vi "RS232 - IIC_H3C QSFP+加密.vi"(0 "VISA resource name":refnum<visa-resource-name>="COM1", 1 "Function":T1(ring)=enum."Read From EEPROM1", 2 "Select channel":u32 max=1, 3 "input_psw":u8[](array[numeric])=[48, 97, 57, 122] format="%.0x", 4 "Data to write":u8[](array[numeric])=[1, 2, 3, 4, 5, 6, 7, 76, 117, 120, 115, 104, 97, 114, 101, 32, 83, 90, 32, 32, 32, 32, 32, 32, 0, 0, 9, 58, 88, 88, 88, 88, 88, 45, 88, 88, 88, 88, 32, 32, 32, 32, 32, 32, 69, 32, 32, 32, 0, 0, 0, 0, 0, 56, 56, 56, 56, 56, 56, 56, 56, 56, 56, 32, 32, 32, 32, 32, 32, 48, 56, 48, 51, 51, 0, 0, 0, 0, 0, 46, 46, 46, 46, 46, 46, 46, 46, 46, 46, 32, 105, 50, 99, 32, 116, 101, 115, 116, 105, 110, 103, 45, 45, 45, 45, 45, 32, 99, 111, 109, 112, 108, 101, 116, 101, 100, 32, 97, 110, 100, 32, 115, 117, 99, 99, 101, 115, 115, 102, 117, 108] format="%x", 5 "Error in":errorcluster) -> (12 "3PagesEqual0":bool, 13 "EEPROM read data":string[][](array[string]), 14 "Duplicate VISA resource name":refnum<visa-resource-name>, 15 "Read Data":string, 16 "Data from Read":u8[](array[numeric])=[255, 255, 255, 255, 255, 255, 255, 255, 255, 255, 255, 255, 255, 255, 255, 255, 255, 255, 255, 255, 255, 82, 101, 118, 49, 46, 49, 255, 255, 255, 255, 255, 255, 255, 255, 255, 255, 255, 255, 255, 255, 255, 255, 255, 255, 255, 255, 255, 255, 255, 255, 255, 255, 255, 255, 255, 255, 255, 255, 255, 255, 255, 255, 255, 255, 255, 255, 255, 255, 255, 255, 255, 255, 255, 255, 255, 255, 255, 255, 255, 255, 255, 255, 255, 255, 255, 255, 255, 255, 255, 255, 255, 255, 255, 255, 255, 255, 255, 255, 255, 255, 255, 255, 255, 255, 255, 255, 255, 255, 255, 255, 255, 255, 255, 255, 255, 255, 255, 255, 255, 255, 255, 255, 255, 255, 255, 255, 255, 255, 255, 255, 255, 255, 255, 255, 255, 255, 255, 255, 255, 255, 255, 255, 255, 255, 255, 255, 255, 255, 82, 101, 118, 49, 46, 49, 255, 255, 255, 255, 255, 255, 255, 255, 255, 255, 255, 255, 255, 255, 255, 255, 255, 255, 255, 255, 255, 255, 255, 255, 255, 255, 255, 255, 255, 255, 255, 255, 255, 255, 255, 255, 255, 255, 255, 255, 255, 255, 255, 255, 255, 255, 255, 255, 255, 255, 255, 255, 255, 255, 255, 255, 255, 255, 255, 255, 255, 255, 255, 255, 255, 255, 255, 255, 255, 255, 255, 255, 255, 255, 255, 255, 255, 255, 255, 255, 255, 255, 255, 255, 255, 255, 255, 255, 255, 255, 255, 255, 255, 255, 255, 255, 255, 255, 255, 255, 255, 255] format="%x", 17 "Message":string, 18 "status":bool=TRUE, 19 "error out":errorcluster={"status"=FALSE, "code"=1073676294, "source"="RS232 - IIC_H3C QSFP+加密.vi中的VISA读取"})   [LabVIEW 2011]
uses:
  <vilib>/Instr/_visa.llb/VISA Configure Serial Port (Instr).vi
panel:
  out "bools":bool[](array[boolean])
  out "x = y?":bool
  out "arrya":u8[][](array[numeric]) format="%.0x"
  in  "Mode":u32(ring) items=["0~EasyI2C", "1~TimingI2C"]
  # "RS232-I2C Writting and Reading"
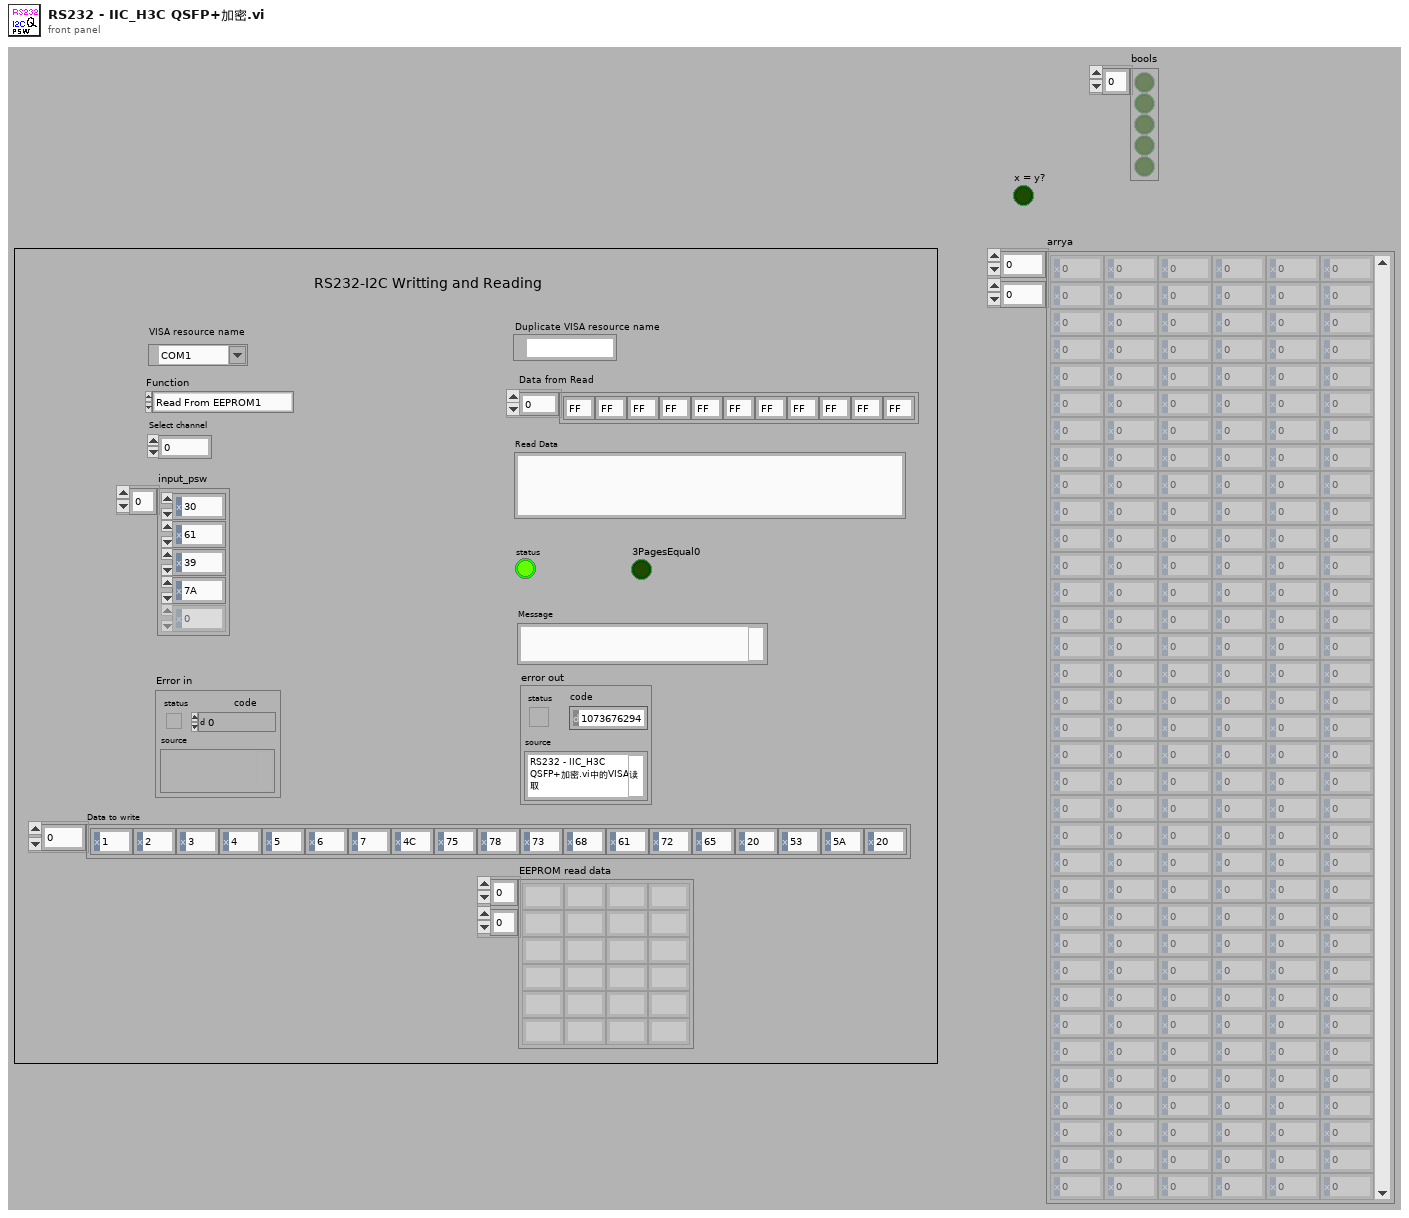
[diagram p1: front panel]
types:
  T1 = enum16{"Write to EEPROM", "Read From EEPROM", "Read From EEPROM1"}
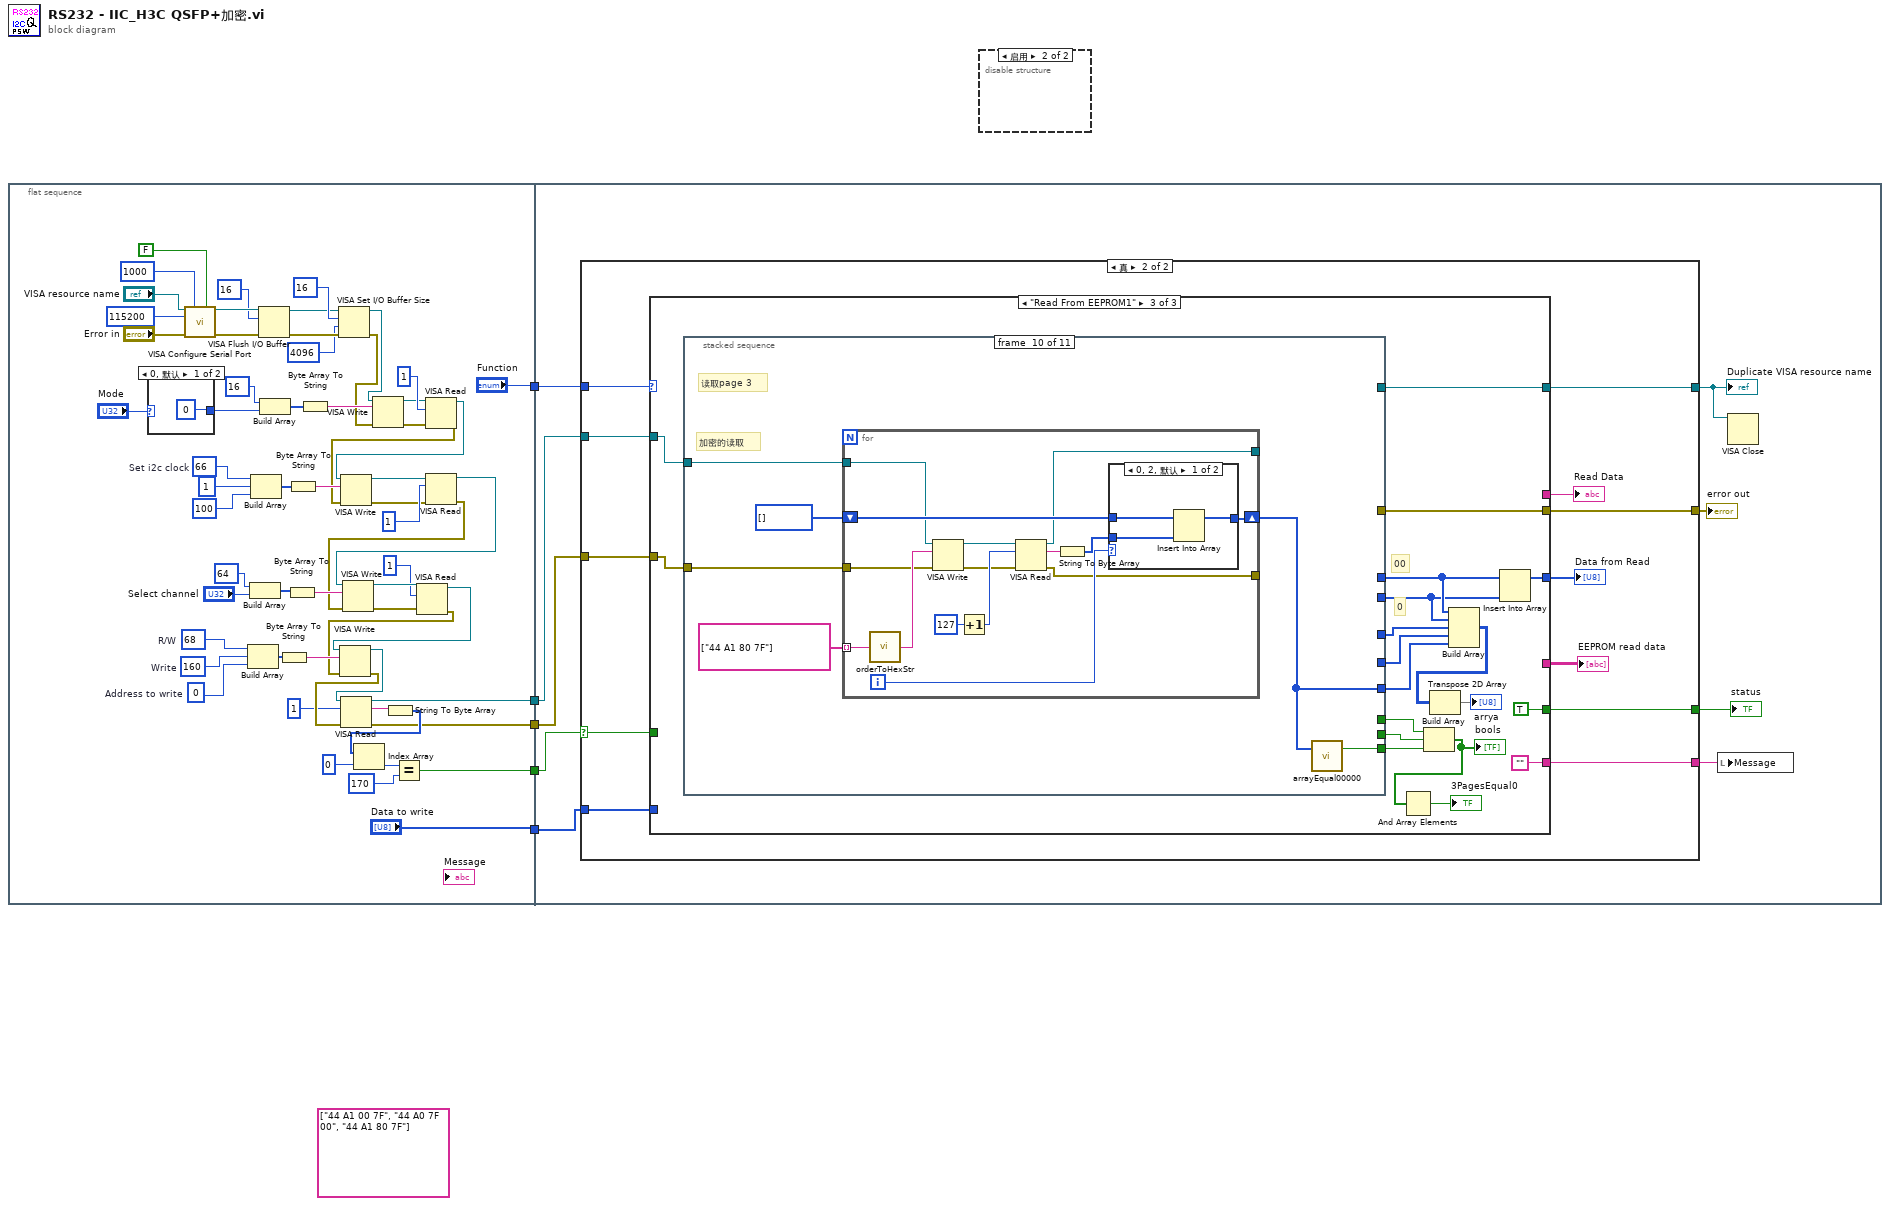
[diagram p0: block diagram]
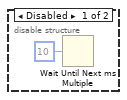
[diagram p2: hidden frame]
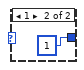
[diagram p3: hidden frame]
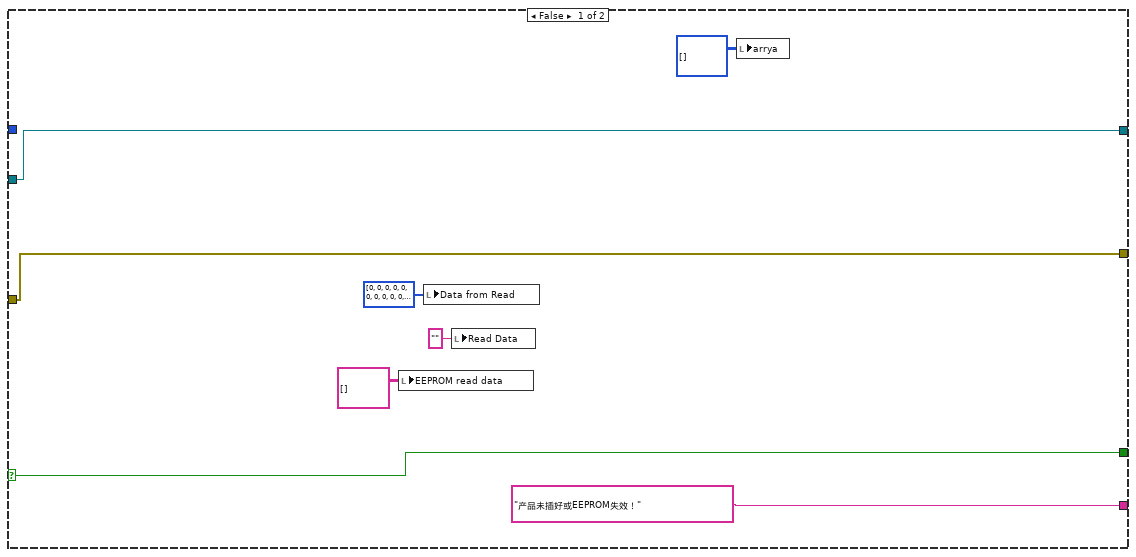
[diagram p4: hidden frame]
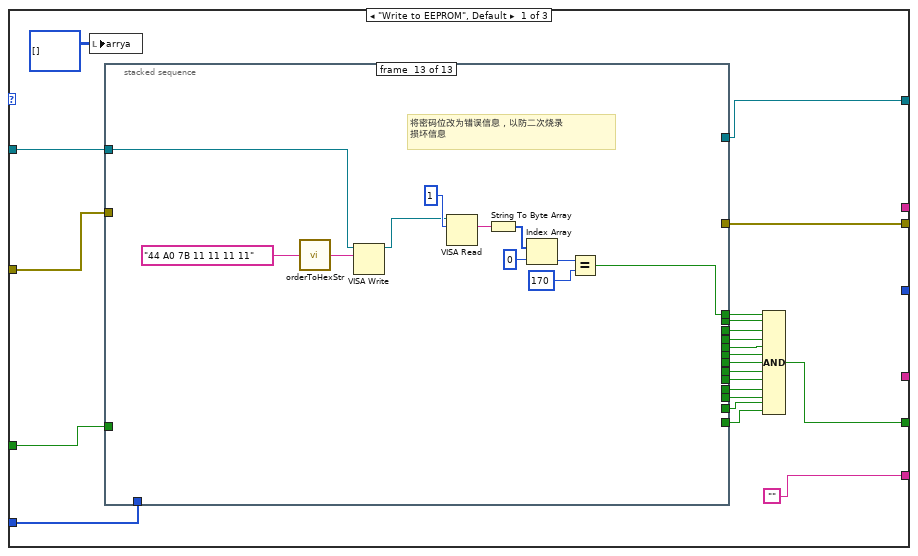
[diagram p5: hidden frame]
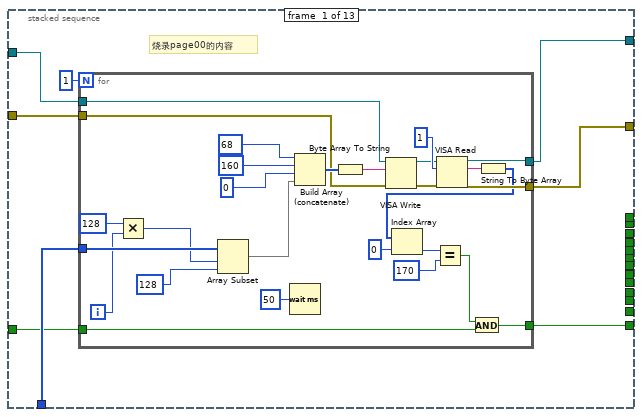
[diagram p6: hidden frame]
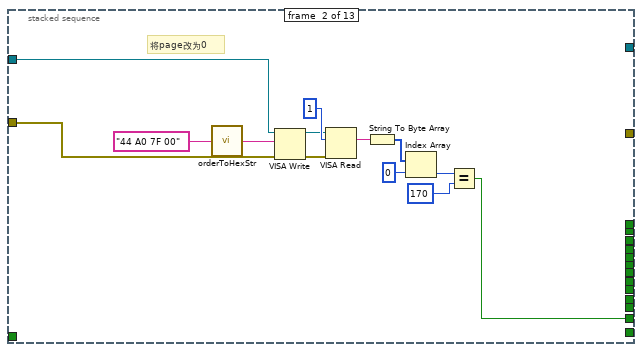
[diagram p7: hidden frame]
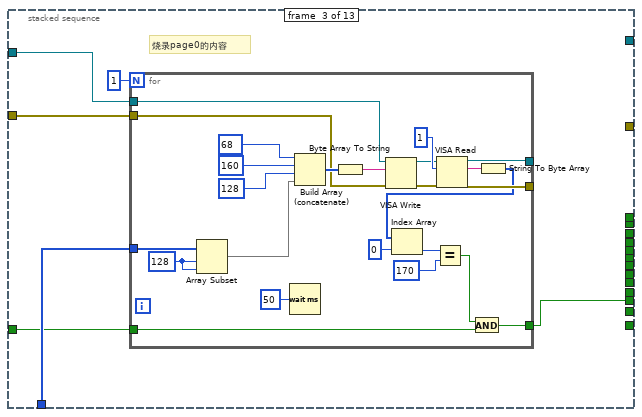
[diagram p8: hidden frame]
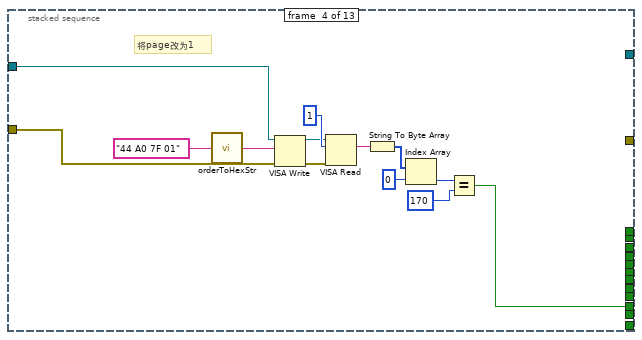
[diagram p9: hidden frame]
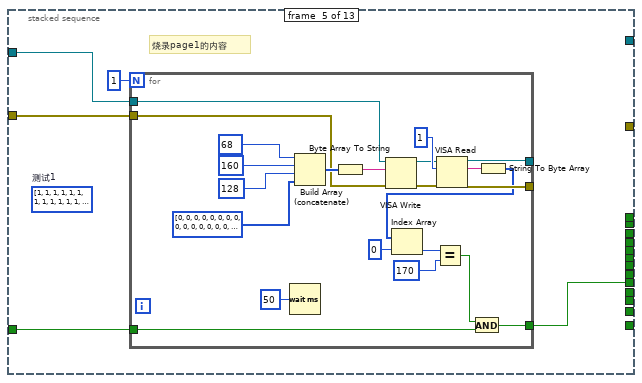
[diagram p10: hidden frame]
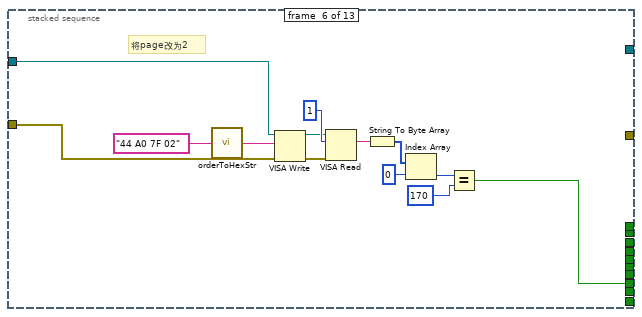
[diagram p11: hidden frame]
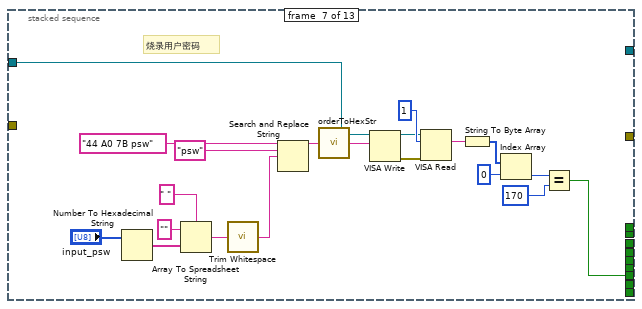
[diagram p12: hidden frame]
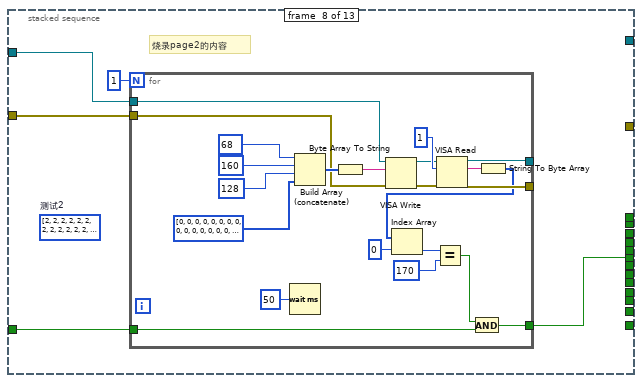
[diagram p13: hidden frame]
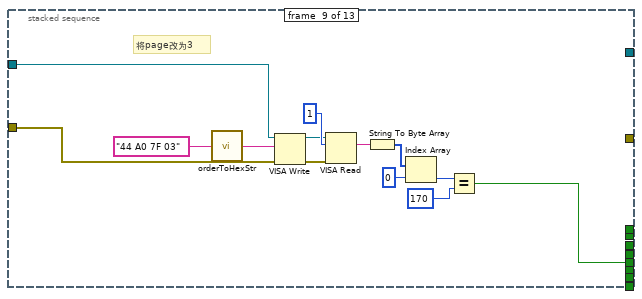
[diagram p14: hidden frame]
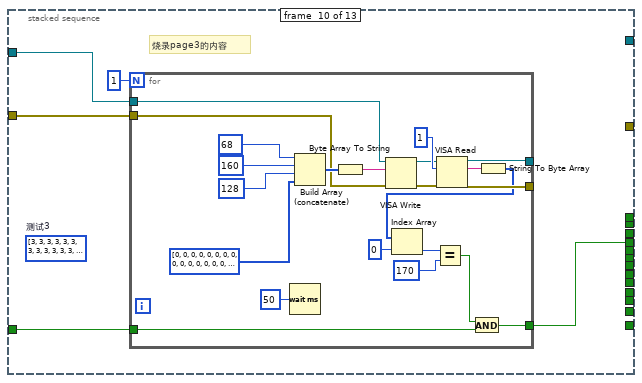
[diagram p15: hidden frame]
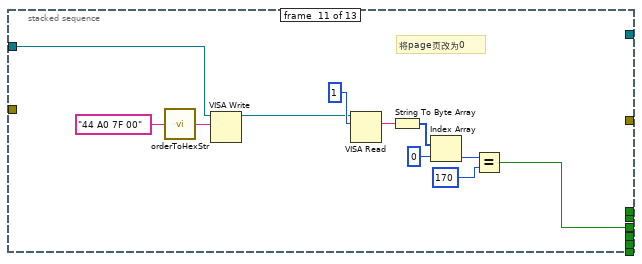
[diagram p16: hidden frame]
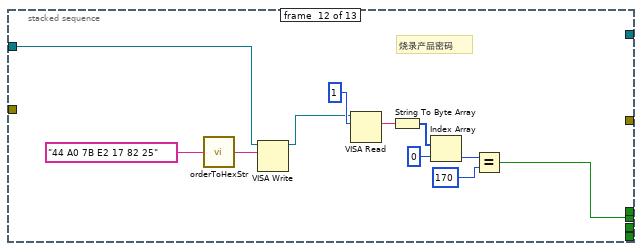
[diagram p17: hidden frame]
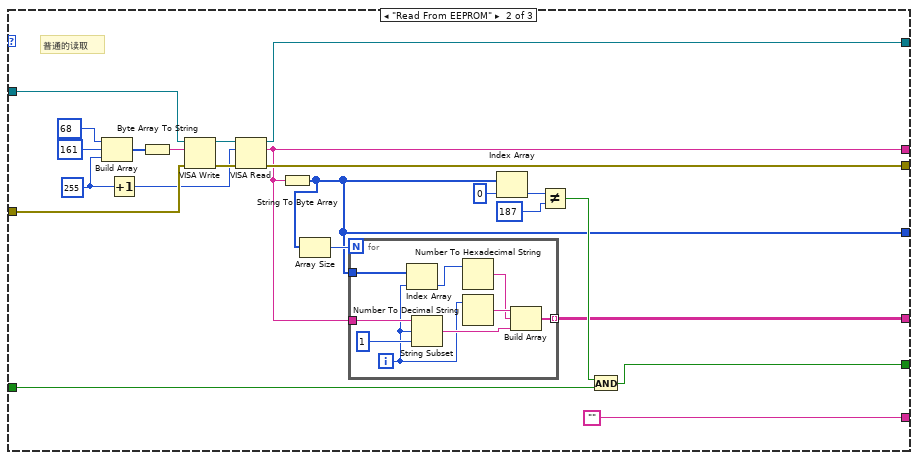
[diagram p18: hidden frame]
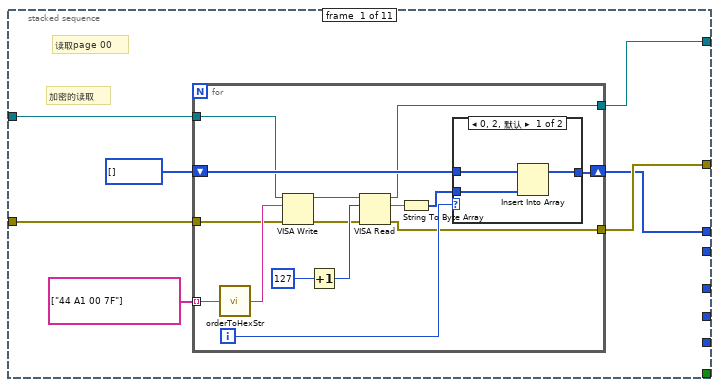
[diagram p19: hidden frame]
diagram:
  (unwired) string[] ["44 A1 00 7F", "44 A0 7F 00", "44 A1 80 7F"]
  n1 = flat-sequence {
    tunnel: [w27] -> w5
    tunnel: [w26] -> w4
    tunnel: [w25] -> w3
    tunnel: ["Function"] -> w2
    tunnel: ["Data to write"] -> w1
    tunnel: w5 -> [w77]
    tunnel: w4 -> [w76]
    tunnel: w3 -> [w75]
    tunnel: w2 -> [w74]
    tunnel: w1 -> [w73]
    frame #0 {
      w31 = u32 0  # Address to write
      w35 = u32 160  # Write
      w33 = u32 68  # R/W
      w48 = u32 66  # Set i2c clock
      n2 = case shown="0, 默认" "Mode" {
        tunnel: [u32 0 ("channel") u32 1 ("channel")] -> w54
        frame 0, Default {
        }
        frame 1 {
        }
      }
      n3 = call-poly "VISA Configure Serial Port"("VISA resource name"="VISA resource name", "timeout (10sec)"=u32 1000 ("timeout"), "Enable Termination\nChar (T)"=FALSE ("Enable Termination\nChar (T)"), "baud rate (9600)"=u32 115200 ("baud rate"), "error in (no error)"="Error in") -> ("VISA resource name out"=w66:refnum<visa-resource-name>, "error out"=w41:errorcluster)  [unwired: 9 in]
      n4 = Build Array(w33, w35, w31) -> (w34:u32[])
      n5 = Build Array(u32 64 ("size (0)"), "Select channel") -> (w52:u32[])
      n6 = Build Array(w48, u32 1 ("size (0)"), u32 100 ("size (0)")) -> (w47:u32[])
      n7 = VISA Flush I/O Buffer(VISA resource name=w66, mask (16)=u16 16, error in (no error)=w41) -> (VISA resource name out=w63:refnum<visa-resource-name>, error out=w62:errorcluster)
      n8 = Build Array(u32 16 ("size (0)"), w54) -> (w53:u32[])
      n9 = Byte Array To String(unsigned byte array=w34) -> (string=w38:string)
      n10 = Byte Array To String(unsigned byte array=w52) -> (string=w44:string)
      n11 = Byte Array To String(unsigned byte array=w47) -> (string=w43:string)
      n12 = Byte Array To String(unsigned byte array=w53) -> (string=w56:string)
      n13 = VISA Set I/O Buffer Size(VISA resource name=w63, mask (16)=u16 16, size (4096)=u32 4096 ("size (0)"), error in (no error)=w62) -> (VISA resource name out=w57:refnum<visa-resource-name>, error out=w40:errorcluster)
      n14 = VISA Write(VISA resource name=w57, write buffer=w56, error in (no error)=w40) -> (VISA resource name out=w19:refnum<visa-resource-name>, error out=w18:errorcluster)  [unwired: 1 out]
      n15 = VISA Read(VISA resource name=w19, byte count=u32 1, error in (no error)=w18) -> (VISA resource name out=w17:refnum<visa-resource-name>, error out=w14:errorcluster)  [unwired: 2 out]
      n16 = VISA Write(VISA resource name=w17, write buffer=w43, error in (no error)=w14) -> (VISA resource name out=w16:refnum<visa-resource-name>, error out=w13:errorcluster)  [unwired: 1 out]
      n17 = VISA Read(VISA resource name=w16, byte count=u32 1, error in (no error)=w13) -> (VISA resource name out=w15:refnum<visa-resource-name>, error out=w12:errorcluster)  [unwired: 2 out]
      n18 = VISA Write(VISA resource name=w15, write buffer=w44, error in (no error)=w12) -> (VISA resource name out=w11:refnum<visa-resource-name>, error out=w10:errorcluster)  [unwired: 1 out]
      n19 = VISA Read(VISA resource name=w11, byte count=u32 1, error in (no error)=w10) -> (VISA resource name out=w8:refnum<visa-resource-name>, error out=w7:errorcluster)  [unwired: 2 out]
      n20 = VISA Write(VISA resource name=w8, write buffer=w38, error in (no error)=w7) -> (VISA resource name out=w32:refnum<visa-resource-name>, error out=w39:errorcluster)  [unwired: 1 out]
      n21 = VISA Read(VISA resource name=w32, byte count=u32 1, error in (no error)=w39) -> (VISA resource name out=w26:refnum<visa-resource-name>, read buffer=w37:string, error out=w25:errorcluster)  [unwired: 1 out]
      n22 = String To Byte Array(string=w37) -> (unsigned byte array=w28:u8[])
      n23 = Index Array(array=w28, index=0) -> (element=w30:u8)
      n24 = Equal?(x=w30, y=u32 170 ("size (0)")) -> (x = y?=w27:bool)
    }
    frame #1 {
      n25 = case shown="真" w77 {
        selector: w77 -> [w82 w93]
        tunnel: w76 -> [w84 w97]
        tunnel: w75 -> [w85 w96]
        tunnel: w74 -> [_ w95]
        tunnel: w73 -> [_ w94]
        tunnel: [w85 w92] -> w70
        tunnel: [w84 w91] -> w69
        tunnel: ["产品未插好或EEPROM失效！" ("message") w90] -> w72
        tunnel: [w82 w86] -> w71
        frame False {
          n26 = local write "EEPROM read data"(string[][] [] ("EEPROM read data")) -> ()
          n27 = local write "Data from Read"(i32[] [0, 0, 0, 0, 0, 0, 0, 0, 0, 0, 0, 0, 0, 0, 0, 0, 0, 0, 0, 0, 0, 0, 0, 0, 0, 0, 0, 0, 0, 0, 0, 0, 0, 0, 0, 0, 0, 0, 0, 0, 0, 0, 0, 0, 0, 0, 0, 0, 0, 0, 0, 0, 0, 0, 0, 0, 0, 0, 0, 0, 0, 0, 0, 0, 0, 0, 0, 0, 0, 0, 0, 0, 0, 0, 0, 0, 0, 0, 0, 0, 0, 0, 0, 0, 0, 0, 0, 0, 0, 0, 0, 0, 0, 0, 0, 0, 0, 0, 0, 0, 0, 0, 0, 0, 0, 0, 0, 0, 0, 0, 0, 0, 0, 0, 0, 0, 0, 0, 0, 0, 0, 0, 0, 0, 0, 0, 0, 0, 0, 0, 0, 0, 0, 0, 0, 0, 0, 0, 0, 0, 0, 0, 0, 0, 0, 0, 0, 0, 0, 0, 0, 0, 0, 0, 0, 0, 0, 0, 0, 0, 0, 0, 0, 0, 0, 0, 0, 0, 0, 0, 0, 0, 0, 0, 0, 0, 0, 0, 0, 0, 0, 0, 0, 0, 0, 0, 0, 0, 0, 0, 0, 0, 0, 0, 0, 0, 0, 0, 0, 0, 0, 0, 0, 0, 0, 0, 0, 0, 0, 0, 0, 0, 0, 0, 0, 0, 0, 0, 0, 0, 0, 0, 0, 0, 0, 0, 0, 0, 0, 0, 0, 0, 0, 0, 0, 0, 0, 0, 0, 0, 0, 0, 0, 0, 0, 0, 0, 0, 0, 0, 0, 0, 0, 0, 0, 0] ("Data from Read")) -> ()
          n28 = local write "Read Data"("" ("Read Data")) -> ()
          n29 = local write "arrya"(u8[][] [] ("arrya")) -> ()
        }
        frame True {
          n30 = case shown="\"Read From EEPROM1\"" w95 {
            tunnel: w97 -> [w119 w393 w419]
            tunnel: w96 -> [w118 w392 w417]
            tunnel: w94 -> [w117 _ _]
            tunnel: [w114 w371 w418] -> w91
            tunnel: [w116 w385 w416] -> w92
            tunnel: w93 -> [w113 w377 _]
            tunnel: ["" ("Message") "" ("Message") "" ("Message")] -> w90
            tunnel: [w101 w375 TRUE] -> w86
            tunnel: [_ w374 _] -> w89
            tunnel: [_ w373 w415] -> w88
            tunnel: [_ w372 _] -> w87
            frame "Write to EEPROM", Default {
              n31 = local write "arrya"(u8[][] [] ("arrya")) -> ()
              n32 = stacked-sequence {
                tunnel: w119 -> [w127 w159 w173 w202 w215 w242 w261 w275 w302 w315 w339 w351 w362]
                tunnel: w118 -> [w126 w158 w172 w201 w214 w241 _ w274 w301 w314 _ _ _]
                tunnel: w117 -> [w125 _ w171 _ _ _ _ _ _ _ _ _ _]
                tunnel: [w123 _ _ _ _ _ _ _ _ _ _ _ _] -> w116
                tunnel: [w124 _ _ _ _ _ _ _ _ _ _ _ _] -> w114
                tunnel: w113 -> [w122 _ w170 _ w213 _ _ w273 _ w313 _ _ _]
                tunnel: [w121 _ _ _ _ _ _ _ _ _ _ _ _] -> w102
                tunnel: [_ w155 _ _ _ _ _ _ _ _ _ _ _] -> w103
                tunnel: [_ _ w168 _ _ _ _ _ _ _ _ _ _] -> w104
                tunnel: [_ _ _ w198 _ _ _ _ _ _ _ _ _] -> w105
                tunnel: [_ _ _ _ w211 _ _ _ _ _ _ _ _] -> w106
                tunnel: [_ _ _ _ _ w238 _ _ _ _ _ _ _] -> w107
                tunnel: [_ _ _ _ _ _ w251 _ _ _ _ _ _] -> w108
                tunnel: [_ _ _ _ _ _ _ w271 _ _ _ _ _] -> w109
                tunnel: [_ _ _ _ _ _ _ _ w298 _ _ _ _] -> w110
                tunnel: [_ _ _ _ _ _ _ _ _ w311 _ _ _] -> w111
                tunnel: [_ _ _ _ _ _ _ _ _ _ w341 _ _] -> w112
                tunnel: [_ _ _ _ _ _ _ _ _ _ _ w349 _] -> w100
                tunnel: [_ _ _ _ _ _ _ _ _ _ _ _ w360] -> w99
                frame #0 {
                  # "烧录page00的内容"
                  n33 = for {
                    N: 1 -> [_]
                    tunnel: w127 -> [w150]
                    tunnel: w125 -> [w133]
                    tunnel: w126 -> [w149]
                    tunnel: [w144] -> w123
                    tunnel: [w142] -> w124
                    tunnel: w122 -> [w137]
                    tunnel: [w136] -> w121
                    i -> [w130]
                    n34 = Multiply(x=128, y=w130) -> (x*y=w128:i32)
                    n35 = Array Subset(array=w133, index=w128, length=128 ("长度")) -> (w131:u8[])
                    n36 = Wait (ms)(milliseconds to wait=u32 50 ("等待时间（毫秒）")) -> ()  [unwired: 1 out]
                    n37 = Build Array (concatenate)(u32 68 ("Write data"), u32 160 ("size (0)"), u32 0 ("元素"), w131) -> (w153:u32[])
                    n38 = Byte Array To String(unsigned byte array=w153) -> (string=w151:string)
                    n39 = VISA Write(VISA resource name=w150, write buffer=w151, error in (no error)=w149) -> (VISA resource name out=w145:refnum<visa-resource-name>, error out=w143:errorcluster)  [unwired: 1 out]
                    n40 = VISA Read(VISA resource name=w145, byte count=u32 1, error in (no error)=w143) -> (VISA resource name out=w142:refnum<visa-resource-name>, read buffer=w141:string, error out=w144:errorcluster)  [unwired: 1 out]
                    n41 = String To Byte Array(string=w141) -> (unsigned byte array=w140:u8[])
                    n42 = Index Array(array=w140, index=0) -> (element=w139:u8)
                    n43 = Equal?(x=w139, y=u32 170 ("size (0)")) -> (x = y?=w138:bool)
                    n44 = And(x=w138, y=w137) -> (x .and. y?=w136:bool)
                  }
                }
                frame #1 {
                  # "将page改为0"
                  n45 = call "orderToHexStr.vi"("I"="44 A0 7F 00") -> ("O"=w156:string)
                  n46 = VISA Write(VISA resource name=w159, write buffer=w156, error in (no error)=w158) -> (VISA resource name out=w164:refnum<visa-resource-name>, error out=w163:errorcluster)  [unwired: 1 out]
                  n47 = VISA Read(VISA resource name=w164, byte count=u32 1, error in (no error)=w163) -> (read buffer=w162:string)  [unwired: 3 out]
                  n48 = String To Byte Array(string=w162) -> (unsigned byte array=w161:u8[])
                  n49 = Index Array(array=w161, index=0) -> (element=w160:u8)
                  n50 = Equal?(x=w160, y=u32 170 ("size (0)")) -> (x = y?=w155:bool)
                }
                frame #2 {
                  # "烧录page0的内容"
                  n51 = for {
                    N: 1 -> [_]
                    tunnel: w173 -> [w193]
                    tunnel: w171 -> [w176]
                    tunnel: w172 -> [w192]
                    tunnel: [w187] -> _
                    tunnel: [w185] -> _
                    tunnel: w170 -> [w180]
                    tunnel: [w179] -> w168
                    w175 = 128 ("索引")
                    n52 = Array Subset(array=w176, index=w175, length=w175) -> (w174:u8[])
                    n53 = Wait (ms)(milliseconds to wait=u32 50 ("等待时间（毫秒）")) -> ()  [unwired: 1 out]
                    n54 = Build Array (concatenate)(u8 68 ("Write data"), u8 160 ("size (0)"), u8 128 ("元素"), w174) -> (w196:u8[])
                    n55 = Byte Array To String(unsigned byte array=w196) -> (string=w194:string)
                    n56 = VISA Write(VISA resource name=w193, write buffer=w194, error in (no error)=w192) -> (VISA resource name out=w188:refnum<visa-resource-name>, error out=w186:errorcluster)  [unwired: 1 out]
                    n57 = VISA Read(VISA resource name=w188, byte count=u32 1, error in (no error)=w186) -> (VISA resource name out=w185:refnum<visa-resource-name>, read buffer=w184:string, error out=w187:errorcluster)  [unwired: 1 out]
                    n58 = String To Byte Array(string=w184) -> (unsigned byte array=w183:u8[])
                    n59 = Index Array(array=w183, index=0) -> (element=w182:u8)
                    n60 = Equal?(x=w182, y=u32 170 ("size (0)")) -> (x = y?=w181:bool)
                    n61 = And(x=w181, y=w180) -> (x .and. y?=w179:bool)
                  }
                }
                frame #3 {
                  # "将page改为1"
                  n62 = call "orderToHexStr.vi"("I"="44 A0 7F 01") -> ("O"=w199:string)
                  n63 = VISA Write(VISA resource name=w202, write buffer=w199, error in (no error)=w201) -> (VISA resource name out=w207:refnum<visa-resource-name>, error out=w206:errorcluster)  [unwired: 1 out]
                  n64 = VISA Read(VISA resource name=w207, byte count=u32 1, error in (no error)=w206) -> (read buffer=w205:string)  [unwired: 3 out]
                  n65 = String To Byte Array(string=w205) -> (unsigned byte array=w204:u8[])
                  n66 = Index Array(array=w204, index=0) -> (element=w203:u8)
                  n67 = Equal?(x=w203, y=u32 170 ("size (0)")) -> (x = y?=w198:bool)
                }
                frame #4 {
                  (unwired) u8[] [1, 1, 1, 1, 1, 1, 1, 1, 1, 1, 1, 1, 1, 1, 1, 1, 1, 1, 1, 1, 1, 1, 1, 1, 1, 1, 1, 1, 1, 1, 1, 1, 1, 1, 1, 1, 1, 1, 1, 1, 1, 1, 1, 1, 1, 1, 1, 1, 1, 1, 1, 1, 1, 1, 1, 1, 1, 1, 1, 1, 1, 1, 1, 1, 1, 1, 1, 1, 1, 1, 1, 1, 1, 1, 1, 1, 1, 1, 1, 1, 1, 1, 1, 1, 1, 1, 1, 1, 1, 1, 1, 1, 1, 1, 1, 1, 1, 1, 1, 1, 1, 1, 1, 1, 1, 1, 1, 1, 1, 1, 1, 1, 1, 1, 1, 1, 1, 1, 1, 1, 1, 1, 1, 1, 1, 1, 1, 1]  # 测试1
                  # "烧录page1的内容"
                  n68 = for {
                    N: 1 -> [_]
                    tunnel: w215 -> [w233]
                    tunnel: w214 -> [w232]
                    tunnel: [w227] -> _
                    tunnel: [w225] -> _
                    tunnel: w213 -> [w220]
                    tunnel: [w219] -> w211
                    n69 = Wait (ms)(milliseconds to wait=u32 50 ("等待时间（毫秒）")) -> ()  [unwired: 1 out]
                    n70 = Build Array (concatenate)(u8 68 ("Write data"), u8 160 ("size (0)"), u8 128 ("元素"), u8[] [0, 0, 0, 0, 0, 0, 0, 0, 0, 0, 0, 0, 0, 0, 0, 0, 0, 0, 0, 0, 0, 0, 0, 0, 0, 0, 0, 0, 0, 0, 0, 0, 0, 0, 0, 0, 0, 0, 0, 0, 0, 0, 0, 0, 0, 0, 0, 0, 0, 0, 0, 0, 0, 0, 0, 0, 0, 0, 0, 0, 0, 0, 0, 0, 0, 0, 0, 0, 0, 0, 0, 0, 0, 0, 0, 0, 0, 0, 0, 0, 0, 0, 0, 0, 0, 0, 0, 0, 0, 0, 0, 0, 0, 0, 0, 0, 0, 0, 0, 0, 0, 0, 0, 0, 0, 0, 0, 0, 0, 0, 0, 0, 0, 0, 0, 0, 0, 0, 0, 0, 0, 0, 0, 0, 0, 0, 0, 0]) -> (w236:u8[])
                    n71 = Byte Array To String(unsigned byte array=w236) -> (string=w234:string)
                    n72 = VISA Write(VISA resource name=w233, write buffer=w234, error in (no error)=w232) -> (VISA resource name out=w228:refnum<visa-resource-name>, error out=w226:errorcluster)  [unwired: 1 out]
                    n73 = VISA Read(VISA resource name=w228, byte count=u32 1, error in (no error)=w226) -> (VISA resource name out=w225:refnum<visa-resource-name>, read buffer=w224:string, error out=w227:errorcluster)  [unwired: 1 out]
                    n74 = String To Byte Array(string=w224) -> (unsigned byte array=w223:u8[])
                    n75 = Index Array(array=w223, index=0) -> (element=w222:u8)
                    n76 = Equal?(x=w222, y=u32 170 ("size (0)")) -> (x = y?=w221:bool)
                    n77 = And(x=w221, y=w220) -> (x .and. y?=w219:bool)
                  }
                }
                frame #5 {
                  # "将page改为2"
                  n78 = call "orderToHexStr.vi"("I"="44 A0 7F 02") -> ("O"=w239:string)
                  n79 = VISA Write(VISA resource name=w242, write buffer=w239, error in (no error)=w241) -> (VISA resource name out=w247:refnum<visa-resource-name>, error out=w246:errorcluster)  [unwired: 1 out]
                  n80 = VISA Read(VISA resource name=w247, byte count=u32 1, error in (no error)=w246) -> (read buffer=w245:string)  [unwired: 3 out]
                  n81 = String To Byte Array(string=w245) -> (unsigned byte array=w244:u8[])
                  n82 = Index Array(array=w244, index=0) -> (element=w243:u8)
                  n83 = Equal?(x=w243, y=u32 170 ("size (0)")) -> (x = y?=w238:bool)
                }
                frame #6 {
                  # "烧录用户密码"
                  n84 = Number To Hexadecimal String(2:"input_psw") -> (0:w258:string[])  [unwired: 1 in]
                  n85 = Array To Spreadsheet String(delimiter (Tab)=" " ("分隔符(Tab)"), array=w258, 3:"" ("格式字符串")) -> (spreadsheet string=w257:string)
                  n86 = call <vilib>:"Trim Whitespace.vi"("string"=w257) -> ("trimmed string"=w253:string)  [unwired: 1 in]
                  n87 = Search and Replace String(input string="44 A0 7B psw", search string="psw" ("搜索字符串"), replace string=w253) -> (result string=w252:string)  [unwired: 5 in, 3 out]
                  n88 = call "orderToHexStr.vi"("I"=w252) -> ("O"=w262:string)
                  n89 = VISA Write(VISA resource name=w261, write buffer=w262) -> (VISA resource name out=w267:refnum<visa-resource-name>, error out=w266:errorcluster)  [unwired: 1 in, 1 out]
                  n90 = VISA Read(VISA resource name=w267, byte count=u32 1, error in (no error)=w266) -> (read buffer=w265:string)  [unwired: 3 out]
                  n91 = String To Byte Array(string=w265) -> (unsigned byte array=w264:u8[])
                  n92 = Index Array(array=w264, index=0) -> (element=w263:u8)
                  n93 = Equal?(x=w263, y=u32 170 ("size (0)")) -> (x = y?=w251:bool)
                }
                frame #7 {
                  (unwired) u8[] [2, 2, 2, 2, 2, 2, 2, 2, 2, 2, 2, 2, 2, 2, 2, 2, 2, 2, 2, 2, 2, 2, 2, 2, 2, 2, 2, 2, 2, 2, 2, 2, 2, 2, 2, 2, 2, 2, 2, 2, 2, 2, 2, 2, 2, 2, 2, 2, 2, 2, 2, 2, 2, 2, 2, 2, 2, 2, 2, 2, 2, 2, 2, 2, 2, 2, 2, 2, 2, 2, 2, 2, 2, 2, 2, 2, 2, 2, 2, 2, 2, 2, 2, 2, 2, 2, 2, 2, 2, 2, 2, 2, 2, 2, 2, 2, 2, 2, 2, 2, 2, 2, 2, 2, 2, 2, 2, 2, 2, 2, 2, 2, 2, 2, 2, 2, 2, 2, 2, 2, 2, 2, 2, 2, 2, 2, 2, 2]  # 测试2
                  # "烧录page2的内容"
                  n94 = for {
                    N: 1 -> [_]
                    tunnel: w275 -> [w293]
                    tunnel: w274 -> [w292]
                    tunnel: [w287] -> _
                    tunnel: [w285] -> _
                    tunnel: w273 -> [w280]
                    tunnel: [w279] -> w271
                    n95 = Wait (ms)(milliseconds to wait=u32 50 ("等待时间（毫秒）")) -> ()  [unwired: 1 out]
                    n96 = Build Array (concatenate)(u8 68 ("Write data"), u8 160 ("size (0)"), u8 128 ("元素"), u8[] [0, 0, 0, 0, 0, 0, 0, 0, 0, 0, 0, 0, 0, 0, 0, 0, 0, 0, 0, 0, 0, 0, 0, 0, 0, 0, 0, 0, 0, 0, 0, 0, 0, 0, 0, 0, 0, 0, 0, 0, 0, 0, 0, 0, 0, 0, 0, 0, 0, 0, 0, 0, 0, 0, 0, 0, 0, 0, 0, 0, 0, 0, 0, 0, 0, 0, 0, 0, 0, 0, 0, 0, 0, 0, 0, 0, 0, 0, 0, 0, 0, 0, 0, 0, 0, 0, 0, 0, 0, 0, 0, 0, 0, 0, 0, 0, 0, 0, 0, 0, 0, 0, 0, 0, 0, 0, 0, 0, 0, 0, 0, 0, 0, 0, 0, 0, 0, 0, 0, 0, 0, 0, 0, 0, 0, 0, 0, 0]) -> (w296:u8[])
                    n97 = Byte Array To String(unsigned byte array=w296) -> (string=w294:string)
                    n98 = VISA Write(VISA resource name=w293, write buffer=w294, error in (no error)=w292) -> (VISA resource name out=w288:refnum<visa-resource-name>, error out=w286:errorcluster)  [unwired: 1 out]
                    n99 = VISA Read(VISA resource name=w288, byte count=u32 1, error in (no error)=w286) -> (VISA resource name out=w285:refnum<visa-resource-name>, read buffer=w284:string, error out=w287:errorcluster)  [unwired: 1 out]
                    n100 = String To Byte Array(string=w284) -> (unsigned byte array=w283:u8[])
                    n101 = Index Array(array=w283, index=0) -> (element=w282:u8)
                    n102 = Equal?(x=w282, y=u32 170 ("size (0)")) -> (x = y?=w281:bool)
                    n103 = And(x=w281, y=w280) -> (x .and. y?=w279:bool)
                  }
                }
                frame #8 {
                  # "将page改为3"
                  n104 = call "orderToHexStr.vi"("I"="44 A0 7F 03") -> ("O"=w299:string)
                  n105 = VISA Write(VISA resource name=w302, write buffer=w299, error in (no error)=w301) -> (VISA resource name out=w307:refnum<visa-resource-name>, error out=w306:errorcluster)  [unwired: 1 out]
                  n106 = VISA Read(VISA resource name=w307, byte count=u32 1, error in (no error)=w306) -> (read buffer=w305:string)  [unwired: 3 out]
                  n107 = String To Byte Array(string=w305) -> (unsigned byte array=w304:u8[])
                  n108 = Index Array(array=w304, index=0) -> (element=w303:u8)
                  n109 = Equal?(x=w303, y=u32 170 ("size (0)")) -> (x = y?=w298:bool)
                }
                frame #9 {
                  (unwired) u8[] [3, 3, 3, 3, 3, 3, 3, 3, 3, 3, 3, 3, 3, 3, 3, 3, 3, 3, 3, 3, 3, 3, 3, 3, 3, 3, 3, 3, 3, 3, 3, 3, 3, 3, 3, 3, 3, 3, 3, 3, 3, 3, 3, 3, 3, 3, 3, 3, 3, 3, 3, 3, 3, 3, 3, 3, 3, 3, 3, 3, 3, 3, 3, 3, 3, 3, 3, 3, 3, 3, 3, 3, 3, 3, 3, 3, 3, 3, 3, 3, 3, 3, 3, 3, 3, 3, 3, 3, 3, 3, 3, 3, 3, 3, 3, 3, 3, 3, 3, 3, 3, 3, 3, 3, 3, 3, 3, 3, 3, 3, 3, 3, 3, 3, 3, 3, 3, 3, 3, 3, 3, 3, 3, 3, 3, 3, 3, 3]  # 测试3
                  # "烧录page3的内容"
                  n110 = for {
                    N: 1 -> [_]
                    tunnel: w315 -> [w333]
                    tunnel: w314 -> [w332]
                    tunnel: [w327] -> _
                    tunnel: [w325] -> _
                    tunnel: w313 -> [w320]
                    tunnel: [w319] -> w311
                    n111 = Wait (ms)(milliseconds to wait=u32 50 ("等待时间（毫秒）")) -> ()  [unwired: 1 out]
                    n112 = Build Array (concatenate)(u8 68 ("Write data"), u8 160 ("size (0)"), u8 128 ("元素"), u8[] [0, 0, 0, 0, 0, 0, 0, 0, 0, 0, 0, 0, 0, 0, 0, 0, 0, 0, 0, 0, 0, 0, 0, 0, 0, 0, 0, 0, 0, 0, 0, 0, 0, 0, 0, 0, 0, 0, 0, 0, 0, 0, 0, 0, 0, 0, 0, 0, 0, 0, 0, 0, 0, 0, 0, 0, 0, 0, 0, 0, 0, 0, 0, 0, 0, 0, 0, 0, 0, 0, 0, 0, 0, 0, 0, 0, 0, 0, 0, 0, 0, 0, 0, 0, 0, 0, 0, 0, 0, 0, 0, 0, 0, 0, 0, 0, 0, 0, 0, 0, 0, 0, 0, 0, 0, 0, 0, 0, 0, 0, 0, 0, 0, 0, 0, 0, 0, 0, 0, 0, 0, 0, 0, 0, 0, 0, 0, 0]) -> (w336:u8[])
                    n113 = Byte Array To String(unsigned byte array=w336) -> (string=w334:string)
                    n114 = VISA Write(VISA resource name=w333, write buffer=w334, error in (no error)=w332) -> (VISA resource name out=w328:refnum<visa-resource-name>, error out=w326:errorcluster)  [unwired: 1 out]
                    n115 = VISA Read(VISA resource name=w328, byte count=u32 1, error in (no error)=w326) -> (VISA resource name out=w325:refnum<visa-resource-name>, read buffer=w324:string, error out=w327:errorcluster)  [unwired: 1 out]
                    n116 = String To Byte Array(string=w324) -> (unsigned byte array=w323:u8[])
                    n117 = Index Array(array=w323, index=0) -> (element=w322:u8)
                    n118 = Equal?(x=w322, y=u32 170 ("size (0)")) -> (x = y?=w321:bool)
                    n119 = And(x=w321, y=w320) -> (x .and. y?=w319:bool)
                  }
                }
                frame #10 {
                  # "将page页改为0"
                  n120 = call "orderToHexStr.vi"("I"="44 A0 7F 00") -> ("O"=w342:string)
                  n121 = VISA Write(VISA resource name=w339, write buffer=w342) -> (VISA resource name out=w338:refnum<visa-resource-name>)  [unwired: 1 in, 2 out]
                  n122 = VISA Read(VISA resource name=w338, byte count=u32 1) -> (read buffer=w340:string)  [unwired: 1 in, 3 out]
                  n123 = String To Byte Array(string=w340) -> (unsigned byte array=w345:u8[])
                  n124 = Index Array(array=w345, index=0) -> (element=w344:u8)
                  n125 = Equal?(x=w344, y=u32 170 ("size (0)")) -> (x = y?=w341:bool)
                }
                frame #11 {
                  # "烧录产品密码"
                  n126 = call "orderToHexStr.vi"("I"="44 A0 7B E2 17 82 25") -> ("O"=w353:string)
                  n127 = VISA Write(VISA resource name=w351, write buffer=w353) -> (VISA resource name out=w350:refnum<visa-resource-name>)  [unwired: 1 in, 2 out]
                  n128 = VISA Read(VISA resource name=w350, byte count=u32 1) -> (read buffer=w354:string)  [unwired: 1 in, 3 out]
                  n129 = String To Byte Array(string=w354) -> (unsigned byte array=w356:u8[])
                  n130 = Index Array(array=w356, index=0) -> (element=w355:u8)
                  n131 = Equal?(x=w355, y=u32 170 ("size (0)")) -> (x = y?=w349:bool)
                }
                frame #12 {
                  # "将密码位改为错误信息，以防二次烧录\n损坏信息"
                  n132 = call "orderToHexStr.vi"("I"="44 A0 7B 11 11 11 11") -> ("O"=w364:string)
                  n133 = VISA Write(VISA resource name=w362, write buffer=w364) -> (VISA resource name out=w361:refnum<visa-resource-name>)  [unwired: 1 in, 2 out]
                  n134 = VISA Read(VISA resource name=w361, byte count=u32 1) -> (read buffer=w365:string)  [unwired: 1 in, 3 out]
                  n135 = String To Byte Array(string=w365) -> (unsigned byte array=w367:u8[])
                  n136 = Index Array(array=w367, index=0) -> (element=w366:u8)
                  n137 = Equal?(x=w366, y=u32 170 ("size (0)")) -> (x = y?=w360:bool)
                }
              }
              n138 = Compound Arithmetic op=AND(w99, w100, w112, w111, w110, w109, w108, w107, w106, w105, w104, w103, w102) -> (w101:bool)
            }
            frame "Read From EEPROM" {
              w382 = u32 255 ("size (0)")
              # "普通的读取"
              n139 = Build Array(u32 68 ("Read data"), u32 161 ("size (0)"), w382) -> (w390:u32[])
              n140 = Increment(x=w382) -> (x+1=w381:u32)
              n141 = Byte Array To String(unsigned byte array=w390) -> (string=w388:string)
              n142 = VISA Write(VISA resource name=w393, write buffer=w388, error in (no error)=w392) -> (VISA resource name out=w387:refnum<visa-resource-name>, error out=w386:errorcluster)  [unwired: 1 out]
              n143 = VISA Read(VISA resource name=w387, byte count=w381, error in (no error)=w386) -> (VISA resource name out=w371:refnum<visa-resource-name>, read buffer=w372:string, error out=w385:errorcluster)  [unwired: 1 out]
              n144 = String To Byte Array(string=w372) -> (unsigned byte array=w373:u8[])
              n145 = Array Size(array=w373) -> (size(s)=w383:i32)
              n146 = for {
                N: w383 -> [_]
                tunnel: w373 -> [w402]
                tunnel: w372 -> [w401]
                tunnel: [w394] -> w374 mode=indexing
                i -> [w397]
                n147 = Index Array(array=w402, index=w397) -> (element=w398:u8)
                n148 = String Subset(string=w401, offset (0)=w397, length (rest)=1 ("length (rest)")) -> (substring=w399:string)
                n149 = Number To Hexadecimal String(2:w398) -> (0:w395:string)  [unwired: 1 in]
                n150 = Number To Decimal String(number=w397) -> (decimal integer string=w396:string)  [unwired: 1 in]
                n151 = Build Array(w396, w395, w399) -> (w394:string[])
              }
              n152 = Index Array(array=w373, index=0) -> (element=w378:u8)
              n153 = Not Equal?(x=w378, y=u32 187 ("size (0)")) -> (x != y?=w376:bool)
              n154 = And(x=w376, y=w377) -> (x .and. y?=w375:bool)
            }
            frame "Read From EEPROM1" {
              # "0"
              # "00"
              n155 = stacked-sequence {
                tunnel: w419 -> [w427 w450 w474 w502 w507 w535 w537 w560 w583 w608 w629]
                tunnel: [w426 _ _ _ _ _ _ _ _ _ _] -> w418
                tunnel: w417 -> [w425 w449 w473 w501 w506 w534 _ w559 w582 w607 _]
                tunnel: [w424 _ _ _ _ _ _ _ _ _ _] -> w416
                tunnel: [_ _ w471 _ _ _ _ _ _ _ _] -> w413
                tunnel: [w422 _ _ _ _ _ _ _ _ _ _] -> w414
                tunnel: [_ _ _ _ w504 _ _ _ _ _ _] -> w412
                tunnel: [_ _ _ _ _ _ _ w557 _ _ _] -> w411
                tunnel: [_ _ _ _ _ _ _ _ _ w605 _] -> w410
                tunnel: [_ _ _ _ w503 _ _ _ _ _ _] -> w407
                tunnel: [_ _ _ _ _ _ _ w556 _ _ _] -> w406
                tunnel: [_ _ _ _ _ _ _ _ _ w604 _] -> w405
                frame #0 {
                  # "读取page 00"
                  # "加密的读取"
                  n156 = for {
                    tunnel: string[] ["44 A1 00 7F"] -> [w439] mode=indexing
                    shift-right: [w436] -> w422
                    shift-left: u8[] [] -> [w437]
                    tunnel: w427 -> [w434]
                    tunnel: [w433] -> w426
                    tunnel: w425 -> [w431]
                    tunnel: [w429] -> w424
                    i -> [w438]
                    n157 = call "orderToHexStr.vi"("I"=w439) -> ("O"=w432:string)
                    n158 = VISA Write(VISA resource name=w434, write buffer=w432, error in (no error)=w431) -> (VISA resource name out=w443:refnum<visa-resource-name>, error out=w430:errorcluster)  [unwired: 1 out]
                    n159 = Increment(x=u32 127 ("size (0)")) -> (x+1=w441:u32)
                    n160 = VISA Read(VISA resource name=w443, byte count=w441, error in (no error)=w430) -> (VISA resource name out=w433:refnum<visa-resource-name>, read buffer=w440:string, error out=w429:errorcluster)  [unwired: 1 out]
                    n161 = String To Byte Array(string=w440) -> (unsigned byte array=w435:u8[])
                    n162 = case shown="0, 2, 默认" w438 {
                      tunnel: w437 -> [w446 w447]
                      tunnel: [w444 w447] -> w436
                      tunnel: w435 -> [w445 _]
                      frame 0, 2, Default {
                        n163 = Insert Into Array(array=w446, new element=w445) -> (w444:u8[])  [unwired: 1 in]
                      }
                      frame 1 {
                      }
                    }
                  }
                }
                frame #1 {
                  # "更改page页 为 0"
                  # "加密的读取"
                  n164 = for {
                    tunnel: string[] ["44 A0 7F 00"] -> [w462] mode=indexing
                    shift-right: [w459] -> _
                    shift-left: u8[] [] -> [w460]
                    tunnel: w450 -> [w457]
                    tunnel: [w456] -> _
                    tunnel: w449 -> [w454]
                    tunnel: [w452] -> _
                    i -> [w461]
                    n165 = call "orderToHexStr.vi"("I"=w462) -> ("O"=w455:string)
                    n166 = VISA Write(VISA resource name=w457, write buffer=w455, error in (no error)=w454) -> (VISA resource name out=w466:refnum<visa-resource-name>, error out=w453:errorcluster)  [unwired: 1 out]
                    n167 = Increment(x=u32 127 ("size (0)")) -> (x+1=w464:u32)
                    n168 = VISA Read(VISA resource name=w466, byte count=w464, error in (no error)=w453) -> (VISA resource name out=w456:refnum<visa-resource-name>, read buffer=w463:string, error out=w452:errorcluster)  [unwired: 1 out]
                    n169 = String To Byte Array(string=w463) -> (unsigned byte array=w458:u8[])
                    n170 = case shown="0, 2, 默认" w461 {
                      tunnel: w460 -> [w469 w470]
                      tunnel: [w467 w470] -> w459
                      tunnel: w458 -> [w468 _]
                      frame 0, 2, Default {
                        n171 = Insert Into Array(array=w469, new element=w468) -> (w467:u8[])  [unwired: 1 in]
                      }
                      frame 1 {
                      }
                    }
                  }
                }
                frame #2 {
                  # "读取page 0"
                  # "加密的读取"
                  n172 = for {
                    tunnel: string[] ["44 A1 80 7F"] -> [w486] mode=indexing
                    shift-right: [w483] -> w471
                    shift-left: u8[] [] -> [w484]
                    tunnel: w474 -> [w481]
                    tunnel: [w480] -> _
                    tunnel: w473 -> [w478]
                    tunnel: [w476] -> _
                    i -> [w485]
                    n173 = call "orderToHexStr.vi"("I"=w486) -> ("O"=w479:string)
                    n174 = VISA Write(VISA resource name=w481, write buffer=w479, error in (no error)=w478) -> (VISA resource name out=w490:refnum<visa-resource-name>, error out=w477:errorcluster)  [unwired: 1 out]
                    n175 = Increment(x=u32 127 ("size (0)")) -> (x+1=w488:u32)
                    n176 = VISA Read(VISA resource name=w490, byte count=w488, error in (no error)=w477) -> (VISA resource name out=w480:refnum<visa-resource-name>, read buffer=w487:string, error out=w476:errorcluster)  [unwired: 1 out]
                    n177 = String To Byte Array(string=w487) -> (unsigned byte array=w482:u8[])
                    n178 = case shown="0, 2, 默认" w485 {
                      tunnel: w484 -> [w493 w494]
                      tunnel: [w491 w494] -> w483
                      tunnel: w482 -> [w492 _]
                      frame 0, 2, Default {
                        n179 = Insert Into Array(array=w493, new element=w492) -> (w491:u8[])  [unwired: 1 in]
                      }
                      frame 1 {
                      }
                    }
                  }
                }
                frame #3 {
                  # "更改page页 为 1"
                  # "加密的读取"
                  n180 = call "orderToHexStr.vi"("I"="44 A0 7F 01") -> ("O"=w497:string)
                  n181 = VISA Write(VISA resource name=w502, write buffer=w497, error in (no error)=w501) -> (VISA resource name out=w500:refnum<visa-resource-name>, error out=w496:errorcluster)  [unwired: 1 out]
                  n182 = Increment(x=u32 0 ("size (0)")) -> (x+1=w498:u32)
                  n183 = VISA Read(VISA resource name=w500, byte count=w498, error in (no error)=w496) -> ()  [unwired: 4 out]
                }
                frame #4 {
                  # "读取page 1"
                  # "加密的读取"
                  n184 = for {
                    tunnel: string[] ["44 A1 80 7F"] -> [w519] mode=indexing
                    shift-right: [w516] -> w504
                    shift-left: u8[] [] -> [w517]
                    tunnel: w507 -> [w514]
                    tunnel: [w513] -> _
                    tunnel: w506 -> [w511]
                    tunnel: [w509] -> _
                    i -> [w518]
                    n185 = call "orderToHexStr.vi"("I"=w519) -> ("O"=w512:string)
                    n186 = VISA Write(VISA resource name=w514, write buffer=w512, error in (no error)=w511) -> (VISA resource name out=w523:refnum<visa-resource-name>, error out=w510:errorcluster)  [unwired: 1 out]
                    n187 = Increment(x=u32 127 ("size (0)")) -> (x+1=w521:u32)
                    n188 = VISA Read(VISA resource name=w523, byte count=w521, error in (no error)=w510) -> (VISA resource name out=w513:refnum<visa-resource-name>, read buffer=w520:string, error out=w509:errorcluster)  [unwired: 1 out]
                    n189 = String To Byte Array(string=w520) -> (unsigned byte array=w515:u8[])
                    n190 = case shown="0, 2, 默认" w518 {
                      tunnel: w517 -> [w526 w527]
                      tunnel: [w524 w527] -> w516
                      tunnel: w515 -> [w525 _]
                      frame 0, 2, Default {
                        n191 = Insert Into Array(array=w526, new element=w525) -> (w524:u8[])  [unwired: 1 in]
                      }
                      frame 1 {
                      }
                    }
                  }
                  n192 = call "arrayEqual00000.vi"("input_array"=w504) -> ("show_bool_result"=w503:bool)  [unwired: 2 in]
                }
                frame #5 {
                  # "更改page页 为 2"
                  # "加密的读取"
                  n193 = call "orderToHexStr.vi"("I"="44 A0 7F 02") -> ("O"=w530:string)
                  n194 = VISA Write(VISA resource name=w535, write buffer=w530, error in (no error)=w534) -> (VISA resource name out=w533:refnum<visa-resource-name>, error out=w529:errorcluster)  [unwired: 1 out]
                  n195 = Increment(x=u32 0 ("size (0)")) -> (x+1=w531:u32)
                  n196 = VISA Read(VISA resource name=w533, byte count=w531, error in (no error)=w529) -> ()  [unwired: 4 out]
                }
                frame #6 {
                  # "烧录用户密码"
                  # "输入密码以便后面读取page 2的值"
                  n197 = local read "input_psw"() -> (w555:u8[])
                  n198 = Number To Hexadecimal String(2:w555) -> (0:w543:string[])  [unwired: 1 in]
                  n199 = Array To Spreadsheet String(delimiter (Tab)=" " ("分隔符(Tab)"), array=w543, 3:"" ("格式字符串")) -> (spreadsheet string=w542:string)
                  n200 = call <vilib>:"Trim Whitespace.vi"("string"=w542) -> ("trimmed string"=w539:string)  [unwired: 1 in]
                  n201 = Search and Replace String(input string="44 A0 7B psw", search string="psw" ("搜索字符串"), replace string=w539) -> (result string=w538:string)  [unwired: 5 in, 3 out]
                  n202 = call "orderToHexStr.vi"("I"=w538) -> ("O"=w546:string)
                  n203 = VISA Write(VISA resource name=w537, write buffer=w546) -> (VISA resource name out=w551:refnum<visa-resource-name>, error out=w550:errorcluster)  [unwired: 1 in, 1 out]
                  n204 = VISA Read(VISA resource name=w551, byte count=u32 1, error in (no error)=w550) -> (read buffer=w549:string)  [unwired: 3 out]
                  n205 = String To Byte Array(string=w549) -> (unsigned byte array=w548:u8[])
                  n206 = Index Array(array=w548, index=0) -> (element=w547:u8)
                  n207 = Equal?(x=w547, y=u32 170 ("size (0)")) -> (x = y?=→"x = y?":bool)
                }
                frame #7 {
                  # "读取page 2"
                  # "加密的读取"
                  n208 = for {
                    tunnel: string[] ["44 A1 80 7F"] -> [w572] mode=indexing
                    shift-right: [w569] -> w557
                    shift-left: u8[] [] -> [w570]
                    tunnel: w560 -> [w567]
                    tunnel: [w566] -> _
                    tunnel: w559 -> [w564]
                    tunnel: [w562] -> _
                    i -> [w571]
                    n209 = call "orderToHexStr.vi"("I"=w572) -> ("O"=w565:string)
                    n210 = VISA Write(VISA resource name=w567, write buffer=w565, error in (no error)=w564) -> (VISA resource name out=w576:refnum<visa-resource-name>, error out=w563:errorcluster)  [unwired: 1 out]
                    n211 = Increment(x=u32 127 ("size (0)")) -> (x+1=w574:u32)
                    n212 = VISA Read(VISA resource name=w576, byte count=w574, error in (no error)=w563) -> (VISA resource name out=w566:refnum<visa-resource-name>, read buffer=w573:string, error out=w562:errorcluster)  [unwired: 1 out]
                    n213 = String To Byte Array(string=w573) -> (unsigned byte array=w568:u8[])
                    n214 = case shown="0, 2, 默认" w571 {
                      tunnel: w570 -> [w579 w580]
                      tunnel: [w577 w580] -> w569
                      tunnel: w568 -> [w578 _]
                      frame 0, 2, Default {
                        n215 = Insert Into Array(array=w579, new element=w578) -> (w577:u8[])  [unwired: 1 in]
                      }
                      frame 1 {
                      }
                    }
                  }
                  n216 = call "arrayEqual00000.vi"("input_array"=w557) -> ("show_bool_result"=w556:bool)  [unwired: 2 in]
                }
                frame #8 {
                  # "更改page页 为 3"
                  # "加密的读取"
                  n217 = for {
                    tunnel: string[] ["44 A0 7F 03"] -> [w595] mode=indexing
                    shift-right: [w592] -> _
                    shift-left: u8[] [] -> [w593]
                    tunnel: w583 -> [w590]
                    tunnel: [w589] -> _
                    tunnel: w582 -> [w587]
                    tunnel: [w585] -> _
                    i -> [w594]
                    n218 = call "orderToHexStr.vi"("I"=w595) -> ("O"=w588:string)
                    n219 = VISA Write(VISA resource name=w590, write buffer=w588, error in (no error)=w587) -> (VISA resource name out=w599:refnum<visa-resource-name>, error out=w586:errorcluster)  [unwired: 1 out]
                    n220 = Increment(x=u32 127 ("size (0)")) -> (x+1=w597:u32)
                    n221 = VISA Read(VISA resource name=w599, byte count=w597, error in (no error)=w586) -> (VISA resource name out=w589:refnum<visa-resource-name>, read buffer=w596:string, error out=w585:errorcluster)  [unwired: 1 out]
                    n222 = String To Byte Array(string=w596) -> (unsigned byte array=w591:u8[])
                    n223 = case shown="0, 2, 默认" w594 {
                      tunnel: w593 -> [w602 w603]
                      tunnel: [w600 w603] -> w592
                      tunnel: w591 -> [w601 _]
                      frame 0, 2, Default {
                        n224 = Insert Into Array(array=w602, new element=w601) -> (w600:u8[])  [unwired: 1 in]
                      }
                      frame 1 {
                      }
                    }
                  }
                }
                frame #9 {
                  # "读取page 3"
                  # "加密的读取"
                  n225 = for {
                    tunnel: string[] ["44 A1 80 7F"] -> [w620] mode=indexing
                    shift-right: [w617] -> w605
                    shift-left: u8[] [] -> [w618]
                    tunnel: w608 -> [w615]
                    tunnel: [w614] -> _
                    tunnel: w607 -> [w612]
                    tunnel: [w610] -> _
                    i -> [w619]
                    n226 = call "orderToHexStr.vi"("I"=w620) -> ("O"=w613:string)
                    n227 = VISA Write(VISA resource name=w615, write buffer=w613, error in (no error)=w612) -> (VISA resource name out=w624:refnum<visa-resource-name>, error out=w611:errorcluster)  [unwired: 1 out]
                    n228 = Increment(x=u32 127 ("size (0)")) -> (x+1=w622:u32)
                    n229 = VISA Read(VISA resource name=w624, byte count=w622, error in (no error)=w611) -> (VISA resource name out=w614:refnum<visa-resource-name>, read buffer=w621:string, error out=w610:errorcluster)  [unwired: 1 out]
                    n230 = String To Byte Array(string=w621) -> (unsigned byte array=w616:u8[])
                    n231 = case shown="0, 2, 默认" w619 {
                      tunnel: w618 -> [w627 w628]
                      tunnel: [w625 w628] -> w617
                      tunnel: w616 -> [w626 _]
                      frame 0, 2, Default {
                        n232 = Insert Into Array(array=w627, new element=w626) -> (w625:u8[])  [unwired: 1 in]
                      }
                      frame 1 {
                      }
                    }
                  }
                  n233 = call "arrayEqual00000.vi"("input_array"=w605) -> ("show_bool_result"=w604:bool)  [unwired: 2 in]
                }
                frame #10 {
                  # "将密码位改为错误信息，以防二次烧录\n损坏信息"
                  n234 = call "orderToHexStr.vi"("I"="44 A0 7B 11 11 11 11") -> ("O"=w632:string)
                  n235 = VISA Write(VISA resource name=w629, write buffer=w632) -> (VISA resource name out=w630:refnum<visa-resource-name>)  [unwired: 1 in, 2 out]
                  n236 = VISA Read(VISA resource name=w630, byte count=u32 1) -> (read buffer=w633:string)  [unwired: 1 in, 3 out]
                  n237 = String To Byte Array(string=w633) -> (unsigned byte array=w635:u8[])
                  n238 = Index Array(array=w635, index=0) -> (element=w634:u8)
                  n239 = Equal?(x=w634, y=u32 170 ("size (0)")) -> ()  [unwired: 1 out]
                }
              }
              n240 = Build Array(w407, w406, w405) -> (w404:bool[])
              "bools" <- w404
              n241 = And Array Elements(Boolean array=w404) -> (logical AND=→"3PagesEqual0":bool)
              n242 = Build Array(w414, w413, w412, w411, w410) -> (w409:u8[][])
              n243 = Transpose 2D Array(2D array=w409) -> (transposed array=→"arrya":u8[][])
              n244 = Insert Into Array(array=w414, new element=w413) -> (w415:u8[])  [unwired: 1 in]
            }
          }
          "EEPROM read data" <- w89
          "Data from Read" <- w88
          "Read Data" <- w87
        }
      }
      "status" <- w71
      "Duplicate VISA resource name" <- w69
      "error out" <- w70
      n245 = local write "Message"(w72) -> ()
      n246 = VISA Close(VISA resource name=w69) -> ()  [unwired: 1 in, 1 out]
    }
  }
  n247 = disable-structure shown="启用" {
    frame Disabled {
      n248 = Wait Until Next ms Multiple(millisecond multiple=u32 10) -> ()  [unwired: 1 out]
    }
    frame Enabled {
    }
  }
